vi "Read CB humidity.vi"(8 "error in (no error)":errorcluster, 11 "Humidity Bricklet in":refnum<class "Humidity Bricklet.lvclass">) -> (0 "error out":errorcluster, 2 "CB humidity":refnum<user-event>, 3 "Humidity Bricklet out":refnum<class "Humidity Bricklet.lvclass">)   [LabVIEW 2011, in "Tinkerforge.lvlib" / "Humidity Bricklet.lvclass"]
uses:
  Humidity Bricklet.lvclass
  Humidity Bricklet.lvclass/Humidity Bricklet.ctl
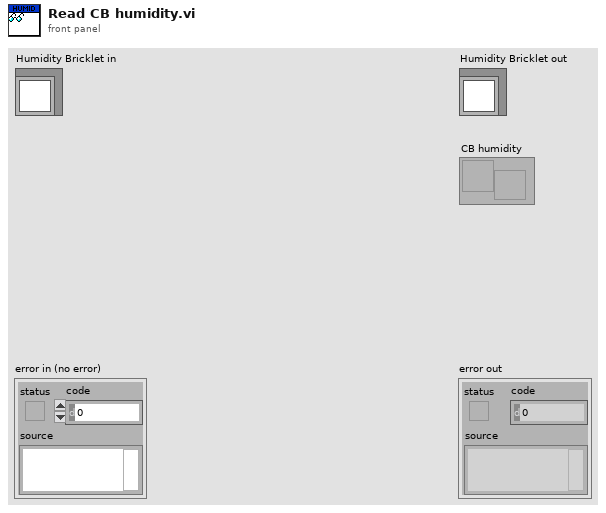
[diagram p1: front panel]
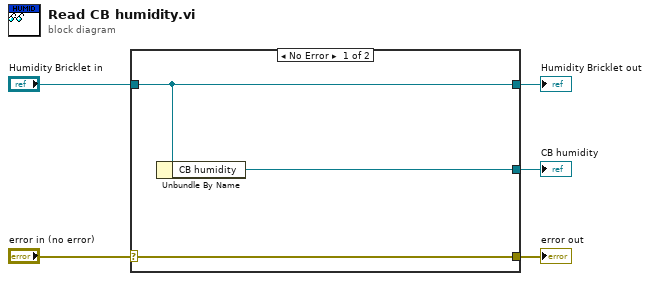
[diagram p0: block diagram]
diagram:
  n1 = case shown="No Error" "error in (no error)" {
    selector: "error in (no error)" -> [w8 w9]
    tunnel: [w8 w9] -> w4
    tunnel: [w7 w10] -> w2
    tunnel: "Humidity Bricklet in" -> [w7 w10]
    tunnel: [w6 _] -> w1
    frame No Error {
      n2 = Unbundle By Name(w7) -> ("CB humidity"=w6:refnum<user-event>)
    }
    frame Error {
    }
  }
  "error out" <- w4
  "Humidity Bricklet out" <- w2
  "CB humidity" <- w1
